vi "I2C_Test.vi"() -> ()   [LabVIEW 2020, in "Rover.lvlib" / "Rover.lvclass"]
uses:
  Rover.lvclass
  <vilib>/MakerHub/LINX/Private/Local IO/LinxI2cWrite.vi
  <vilib>/MakerHub/LINX/Public/Utilities/Check Channel.vi
  <vilib>/MakerHub/LINX/Private/Local IO/Handle Errors.vi
  <vilib>/MakerHub/LINX/Public/Utilities/Open Local.vi
  <vilib>/MakerHub/LINX/Private/Utilties/Generate Error.vi
  <vilib>/MakerHub/LINX/LMH-LINX.lvlib
panel:
  out "Error Out":errorcluster
  in  "stop":bool
  out "C":u8
  in  "Equals":bool
  in  "B":u8
  in  "A":u8
  # "+"
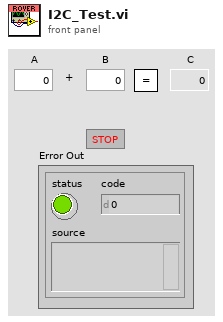
[diagram p1: front panel]
types:
  T1 = typedef "LMH-LINX.lvlib/LINX Ref.ctl" = cluster{"IO":T2, "Interface":T3, "LINX Device Config":T4}
  T2 = typedef "LMH-LINX.lvlib/Platform.ctl" = enum16{"Remote", "Local"}
  T3 = typedef "LMH-LINX.lvlib/Interface.ctl" = enum16{"Serial", "TCP"}
  T4 = typedef "LMH-LINX.lvlib/Device.lvlib/LINX Device Config.ctl" = cluster{"Interface":T3, "COM Port":refnum<visa-resource-name>, "TCP Configuration":T5, "Device Family":u8, "Device ID":u8, "Device Name":string, "TCP Ref":refnum<k5>, "Channels":T6}
  T5 = typedef "LMH-LINX.lvlib/Device.lvlib/TCP Config.ctl" = cluster{"IP Address":string, "Port":u16}
  T6 = typedef "LMH-LINX.lvlib/Channels.ctl" = cluster{"DI":u8[], "DO":u8[], "AI":u8[], "AO":u8[], "PWM":u8[], "QE":u8[], "UART":u8[], "I2C 2":u8[], "SPI":u8[], "CAN":u8[], "Servo":u8[], "AI Ref (V)":dbl, "AI Resolution (Bits)":u8, "AO Ref (V)":dbl, "AO Resolution (Bits)":u8}
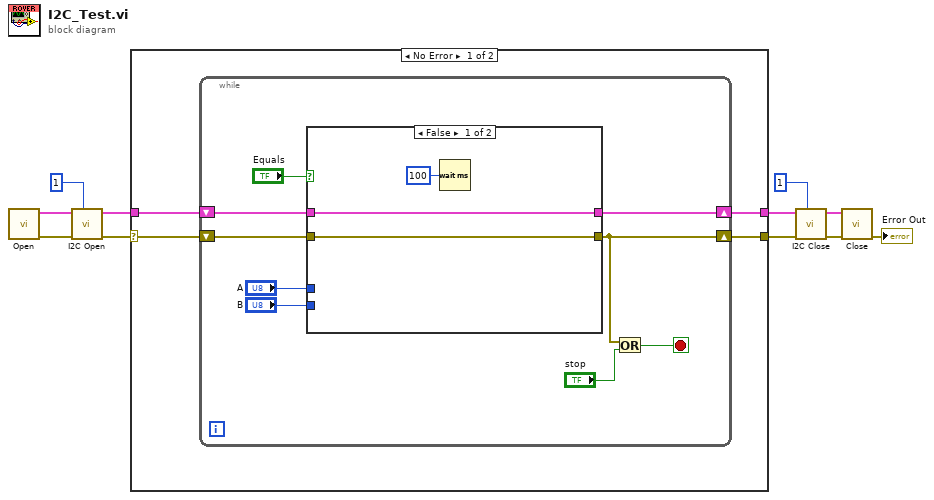
[diagram p0: block diagram]
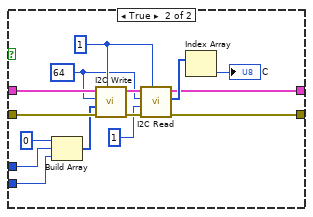
[diagram p2: hidden frame]
diagram:
  n1 = call-poly <vilib>:"Open.vi"() -> ("Error Out"=w10:errorcluster, "LINX Resource"=w11:T1)  [unwired: 9 in, 1 out]
  n2 = call <vilib>:"I2C Open.vi"("I2C Channel (0)"=u8 1, "Error In"=w10, "LINX Resource"=w11) -> ("Error Out"=w8:errorcluster, "LINX Resource"=w7:T1)  [unwired: 7 in]
  n3 = case shown="No Error" w8 {
    selector: w8 -> [w15 w44]
    tunnel: w7 -> [w14 w43]
    tunnel: [w13 w44] -> w5
    tunnel: [w12 w43] -> w6
    frame No Error {
      n4 = while {
        shift-right: [w18] -> w13
        shift-left: w15 -> [w23]
        shift-right: [w19] -> w12
        shift-left: w14 -> [w24]
        stop <- w16 stop-if-true
        n5 = case shown="False" "Equals" {
          tunnel: w24 -> [w26 w42]
          tunnel: w23 -> [w25 w41]
          tunnel: "A" -> [_ w39]
          tunnel: "B" -> [_ w38]
          tunnel: [w26 w29] -> w19
          tunnel: [w25 w28] -> w18
          frame False {
            n6 = Wait (ms)(milliseconds to wait=u32 100) -> ()  [unwired: 1 out]
          }
          frame True {
            w33 = u8 64 ("I2C Slave Address (0)")
            w34 = u8 1 ("I2C Channel")
            n7 = Build Array(u8 0, w39, w38) -> (w37:u8[])
            n8 = call <vilib>:"I2C Write.vi"("I2C Channel"=w34, "Error In"=w41, "Data"=w37, "I2C Slave Address (0)"=w33, "LINX Resource"=w42) -> ("Error Out"=w35:errorcluster, "LINX Resource"=w36:T1)  [unwired: 5 in]
            n9 = call <vilib>:"I2C Read.vi"("I2C Channel"=w34, "Error In"=w35, "Bytes To Read"=u8 1, "I2C Slave Address (0)"=w33, "LINX Resource"=w36) -> ("Error Out"=w28:errorcluster, "Data"=w31:u8[], "LINX Resource"=w29:T1)  [unwired: 4 in]
            n10 = Index Array(array=w31) -> (element=→"C":u8)  [unwired: 1 in]
          }
        }
        n11 = Or(x=w18, y="stop") -> (x .or. y?=w16:bool)
      }
    }
    frame Error {
    }
  }
  n12 = call <vilib>:"I2C Close.vi"("I2C Channel (0)"=u8 1, "Error In"=w5, "LINX Resource"=w6) -> ("Error Out"=w2:errorcluster, "LINX Resource"=w3:T1)  [unwired: 7 in]
  n13 = call <vilib>:"Close.vi"("Error In"=w2, "LINX Resource"=w3) -> ("Error Out"=→"Error Out":errorcluster)  [unwired: 9 in]
